vi "Remove OpenG Tools from llb.vi"(8 "error in (no error)":errorcluster, 11 "Path":path) -> (0 "error out":errorcluster)   [LabVIEW 2019]
uses:
  <vilib>/Utility/libraryn.llb/Librarian File List.ctl
panel:
  out "size(s)":i32
  out "size after":i32
  out "size before":i32
  out "Deleted Files":path[](array[path])
  out "file list":T1 {"LV version" format="%.0x"}
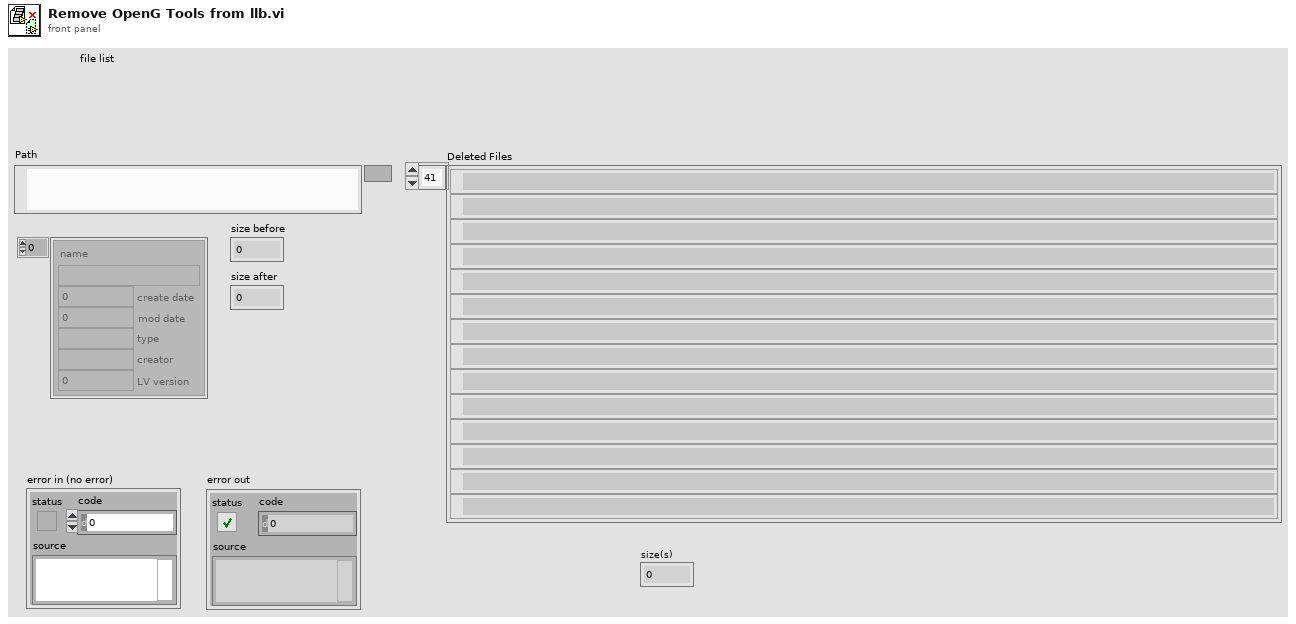
[diagram p1: front panel]
types:
  T1 = typedef "Librarian File List.ctl" = cluster{"name":string, "create date":u32, "mod date":u32, "type":string, "creator":string, "LV version":i32}[]
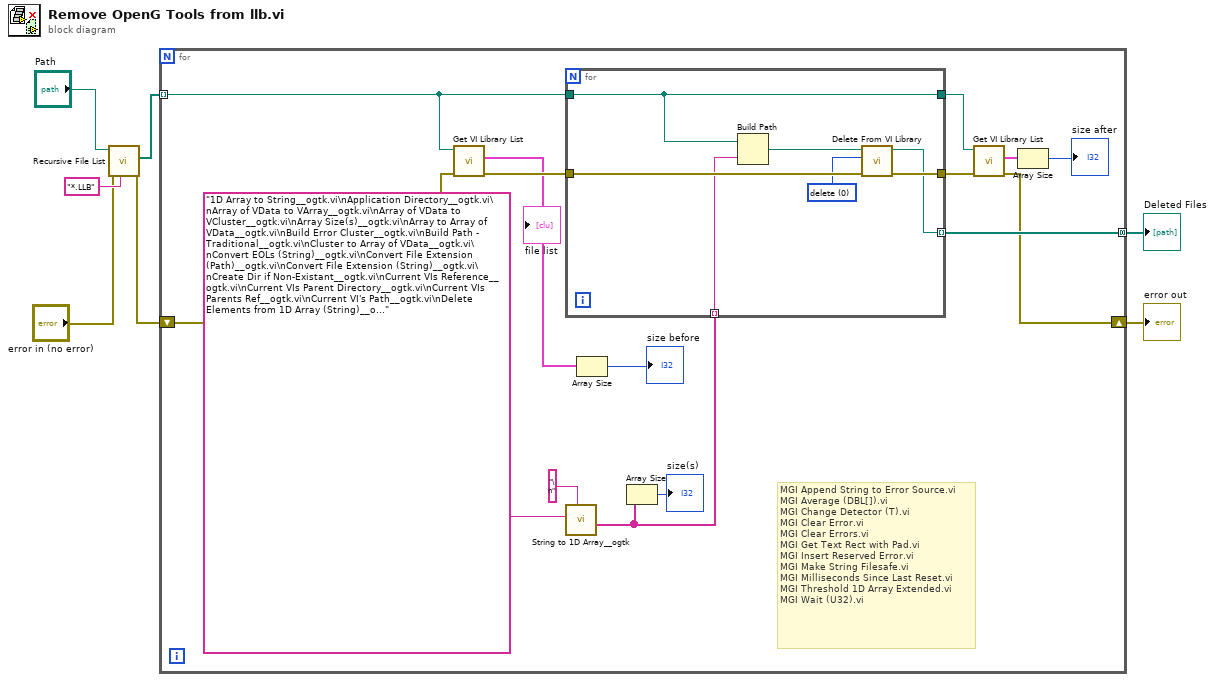
[diagram p0: block diagram]
diagram:
  n1 = call <vilib>:"Recursive File List.vi"("pattern"="*.LLB", "error in (no error)"="error in (no error)", "Folder Path"="Path") -> ("error out"=w2:errorcluster, "All Files in Dir"=w1:path[])  [unwired: 4 in, 3 out]
  n2 = for {
    tunnel: [w21] -> w7 mode=concatenating
    tunnel: w1 -> [w13] mode=indexing
    shift-right: [w14] -> w6
    shift-left: w2 -> [w12]
    # "MGI Append String to Error Source.vi\nMGI Average (DBL[]).vi\nMGI Change Detector (T).vi\nMGI Clear Error.vi\nMGI Clear Errors.vi\nMGI Get Text Rect with Pad.vi\nMGI Insert Reserved Error.vi\nMGI Make String Filesafe.vi\nMGI Milliseconds Since Last Reset.vi\nMGI Threshold 1D Array Extended.vi\nMGI Wait (U32).vi"
    n3 = call <vilib>:"Get VI Library List.vi"("error in (no error)"=w12, "library path"=w13) -> ("error out"=w22:errorcluster, "file list"=w15:T1)  [unwired: 8 in]
    "file list" <- w15
    n4 = call <userlib>:"String to 1D Array__ogtk.vi"("delimiter (Tab)"="\n", "string"="1D Array to String__ogtk.vi\nApplication Directory__ogtk.vi\nArray of VData to VArray__ogtk.vi\nArray of VData to VCluster__ogtk.vi\nArray Size(s)__ogtk.vi\nArray to Array of VData__ogtk.vi\nBuild Error Cluster__ogtk.vi\nBuild Path - Traditional__ogtk.vi\nCluster to Array of VData__ogtk.vi\nConvert EOLs (String)__ogtk.vi\nConvert File Extension (Path)__ogtk.vi\nConvert File Extension (String)__ogtk.vi\nCreate Dir if Non-Existant__ogtk.vi\nCurrent VIs Reference__ogtk.vi\nCurrent VIs Parent Directory__ogtk.vi\nCurrent VIs Parents Ref__ogtk.vi\nCurrent VI's Path__ogtk.vi\nDelete Elements from 1D Array (String)__ogtk.vi\nDelete Elements from 1D Array (DBL)__ogtk.vi\nEncode Section and Key Names__ogtk.vi\nEmpty 2D Array (String)__ogtk.vi\nFile Exists - Scalar__ogtk.vi\nFile Info Record__ogtk.ctl\nFile Info__ogtk.vi\nFilter 1D Array (String)__ogtk.vi\nFormat Numeric Array__ogtk.vi\nFormat Variant Into String__ogtk.vi\nGet Array Element TD__ogtk.vi\nGet Array Element Default Data__ogtk.vi\nGet Array Element TDEnum__ogtk.vi\nGet Data Name from TD__ogtk.vi\nGet Data Name__ogtk.vi\nGet Default Data from TD__ogtk.vi\nGet Element TD from Array TD__ogtk.vi\nGet Header from TD__ogtk.vi\nGet Last PString__ogtk.vi\nGet PString__ogtk.vi\nGet Strings from Enum TD__ogtk.vi\nGet Strings from Enum__ogtk.vi\nGet TDEnum from Data__ogtk.vi\nGet Refnum Type Enum from Data__ogtk.vi\nGet Refnum Type Enum from TD__ogtk.vi\nGet Variant Attributes__ogtk.vi\nGet Waveform Type Enum from Data__ogtk.vi\nGet Waveform Type Enum from TD__ogtk.vi\nIndex 1D Array Elements (DBL)__ogtk.vi\nLVOOP Get Default Object__ogtk.vi\nLVOOP Return Class Name__ogtk.vi\nMulti-line String to Array__ogtk.vi\nParse String with TDs__ogtk.vi\nPeriodic Trigger__ogtk.vi\nRead Key (Variant)__ogtk.vi\nRead Section Cluster__ogtk.vi\nRefnum Subtype Enum__ogtk.ctl\nRemove Duplicates from 1D Array (String)__ogtk.vi\nRemove Duplicates from 1D Array (DBL)__ogtk.vi\nReorder 1D Array2 (DBL)__ogtk.vi\nReorder 1D Array2 (String)__ogtk.vi\nReshape 1D Array__ogtk.vi\nReshape Array to 1D VArray__ogtk.vi\nResolve Timestamp Format__ogtk.vi\nSearch 1D Array (Boolean)__ogtk.vi\nSearch 1D Array (String)__ogtk.vi\nSet Data Name__ogtk.vi\nSet Enum String Value__ogtk.vi\nSort 1D Array (DBL)__ogtk.vi\nSort 1D Array (I32)__ogtk.vi\nSort 1D Array (U32)__ogtk.vi\nSort 2D Array (DBL)__ogtk.vi\nSlice String 1__ogtk.vi\nString to 1D Array__ogtk.vi\nSplit Cluster TD__ogtk.vi\nStrip Path - Traditional__ogtk.vi\nStrip Path Extension - Path__ogtk.vi\nStrip Path Extension - String__ogtk.vi\nStrip Units__ogtk.vi\nTemporary Directory__ogtk.vi\nTrim Whitespace (String)__ogtk.vi\nType Descriptor Enumeration__ogtk.ctl\nType Descriptor Header__ogtk.ctl\nType Descriptor__ogtk.ctl\nValid Path - Traditional__ogtk.vi\nVariant to Header Info__ogtk.vi\nWait (ms)__ogtk.vi\nWaveform Subtype Enum__ogtk.ctl\nMGI Append String to Error Source.vi\nMGI Average (DBL[]).vi\nMGI Change Detector (T).vi\nMGI Clear Error.vi\nMGI Clear Errors.vi\nMGI Get Text Rect with Pad.vi\nMGI Insert Reserved Error.vi\nMGI Make String Filesafe.vi\nMGI Milliseconds Since Last Reset.vi\nMGI Threshold 1D Array Extended.vi\nMGI Wait (U32).vi") -> ("Array of Strings"=w9:string[])  [unwired: 9 in]
    n5 = for {
      tunnel: w13 -> [w25]
      tunnel: w22 -> [w27]
      tunnel: [w26] -> w21 mode=indexing
      tunnel: [w28] -> w17
      tunnel: [w25] -> w16
      tunnel: w9 -> [w24] mode=indexing
      w23 = u16 0 items=["delete", "ask first"] ("delete")
      n6 = Build Path(base path=w25, name or relative path=w24) -> (appended path=w26:path)
      n7 = call <vilib>:"Delete From VI Library.vi"("error in (no error)"=w27, "delete"=w23, "path"=w26) -> ("error out"=w28:errorcluster)  [unwired: 8 in]
    }
    n8 = Array Size(array=w15) -> (size(s)=→"size before":i32)
    n9 = Array Size(array=w9) -> (size(s)=→"size(s)":i32)
    n10 = call <vilib>:"Get VI Library List.vi"("error in (no error)"=w17, "library path"=w16) -> ("error out"=w14:errorcluster, "file list"=w18:T1)  [unwired: 8 in]
    n11 = Array Size(array=w18) -> (size(s)=→"size after":i32)
  }
  "Deleted Files" <- w7
  "error out" <- w6
